vi "Generate Publisher Message Set.vi"(9 "Mediator Enqueuer":refnum<class "Message Enqueuer.lvclass">, 11 "IMediator in":refnum<class "IMediator.lvclass">) -> (1 "Unlock Publication Msg":refnum<class "Unlock Publication Msg.lvclass">, 2 "Lock Publication Msg":refnum<class "Lock Publication Msg.lvclass">, 3 "Publish Msg":refnum<class "Publish Msg.lvclass">)   [LabVIEW 2018, in "MVA Framework.lvlib" / "IMediator.lvlib" / "IMediator.lvclass"]
doc: "生成发布者消息集"
uses:
  IMediator.lvclass
  IMediator Messages/Publish Msg/Publish Msg.lvclass
  IMediator Messages/Lock Publication Msg/Lock Publication Msg.lvclass
  IMediator Messages/Unlock Publication Msg/Unlock Publication Msg.lvclass
  <vilib>/ActorFramework/Message Enqueuer/Message Enqueuer.lvclass
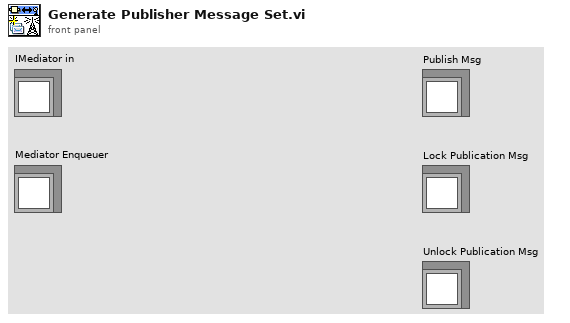
[diagram p1: front panel]
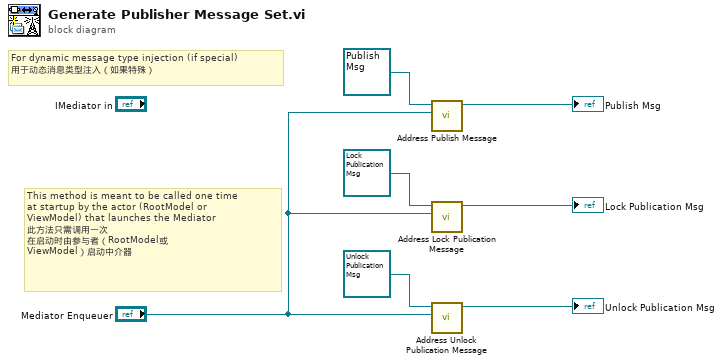
[diagram p0: block diagram]
diagram:
  # "This method is meant to be called one time\nat startup by the actor (RootModel or\nViewModel) that launches the Mediator\n此方法只需调用一次\n在启动时由参与者（RootModel或\nViewModel）启动中介器"
  # "For dynamic message type injection (if special)\n用于动态消息类型注入（如果特殊）"
  n1 = call "Address Publish Message.vi"("Mediator Enqueuer"="Mediator Enqueuer", "Publish Msg in"=refnum<class "Publish Msg.lvclass"> refnum ("Subscribe Msg In")) -> ("Publish Msg out"=→"Publish Msg":refnum<class "Publish Msg.lvclass">)  [unwired: 9 in]
  n2 = call "Address Lock Publication Message.vi"("Mediator Enqueuer"="Mediator Enqueuer", "Lock Publication Msg In"=refnum<class "Lock Publication Msg.lvclass"> refnum ("Unsubscribe Msg In")) -> ("Lock Publication Msg Out"=→"Lock Publication Msg":refnum<class "Lock Publication Msg.lvclass">)  [unwired: 9 in]
  n3 = call "Address Unlock Publication Message.vi"("Mediator Enqueuer"="Mediator Enqueuer", "Unlock Publication Msg In"=refnum<class "Unlock Publication Msg.lvclass"> refnum ("Unsubscribe Msg In")) -> ("Unlock Publication Msg Out"=→"Unlock Publication Msg":refnum<class "Unlock Publication Msg.lvclass">)  [unwired: 9 in]
